vi "RWAllParameters_SRSI.vi"(8 "error in (no error)":errorcluster, 9 "Read/Write":T1(ring), 10 "Parameters In (Variant)":variant[](array[variant]), 11 "Parameters In":T2={"sensitivity"=0.11032028469750889, "Filter"={"Tau (fs)"=9.75e-13, "fwhm (fs)"=3.2551150895140684e-13, "filter gaussian power"=30}, "Poly Fit Order"=4, "N XPW Loop"=3, "Scales Unit"=enum."nm", "Results average"=0, "Spectral filter"={"min"=0.0, "max"=0.0, "Level"=0.0}, "Apodization"={"Auto"=TRUE, "WL min"=6.000000000000001e-07, "WL max"=1.0000000000000002e-06}, "Warning levels"={"Min level"=5000.0, "Max level"=62000.0, "Min contrast"=0.1}, "NormXPW"=FALSE, "DisableChecks"=FALSE, "External\nFund. Spectrum"=FALSE, "XPW factors"={"Optimize"=enum."Never", "Blue Shift Correction"=0.0, "Parasite Amp"=0.0}}) -> (0 "error out":errorcluster, 2 "Parameters Out":variant[](array[variant]), 3 "Parameters Out":T2={"sensitivity"=0.11032028469750889, "Filter"={"Tau (fs)"=9.75e-13, "fwhm (fs)"=3.2551150895140684e-13, "filter gaussian power"=30}, "Poly Fit Order"=4, "N XPW Loop"=3, "Scales Unit"=enum."nm", "Results average"=0, "Spectral filter"={"min"=0.0, "max"=0.0, "Level"=0.0}, "Apodization"={"Auto"=TRUE, "WL min"=6.000000000000001e-07, "WL max"=1.0000000000000002e-06}, "Warning levels"={"Min level"=5000.0, "Max level"=62000.0, "Min contrast"=0.1}, "NormXPW"=FALSE, "DisableChecks"=FALSE, "External\nFund. Spectrum"=FALSE, "XPW factors"={"Optimize"=enum."Never", "Blue Shift Correction"=0.0, "Parasite Amp"=0.0}})   [LabVIEW 2020]
uses:
  SRSI_Parameters.ctl
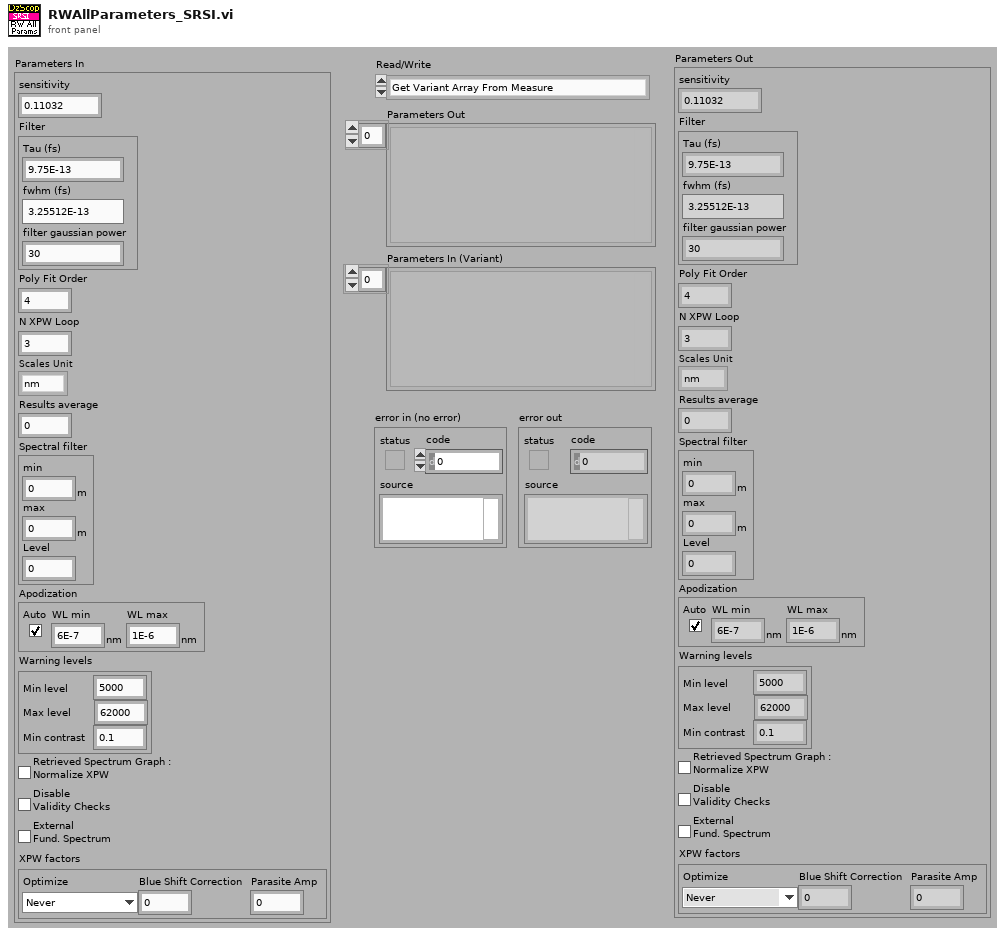
[diagram p1: front panel]
types:
  T1 = enum16{"Get Variant Array From Measure", "Set Measure From Variant Array"}
  T2 = typedef "SRSI_Parameters.ctl" = cluster{"sensitivity":dbl, "Filter":cluster{"Tau (fs)":dbl[unit], "fwhm (fs)":dbl[unit], "filter gaussian power":i32}, "Poly Fit Order":i32, "N XPW Loop":u16, "Scales Unit":enum16{"nm", "THz", "cm^-1"}, "Results average":i32, "Spectral filter":cluster{"min":dbl[unit], "max":dbl[unit], "Level":dbl}, "Apodization":cluster{"Auto":bool, "WL min":dbl[unit], "WL max":dbl[unit]}, "Warning levels":cluster{"Min level":dbl, "Max level":dbl, "Min contrast":dbl}, "NormXPW":bool, "DisableChecks":bool, "External\nFund. Spectrum":bool, "XPW factors":cluster{"Optimize":enum16{"Never", "Once", "Ever"}, "Blue Shift Correction":dbl, "Parasite Amp":dbl}}
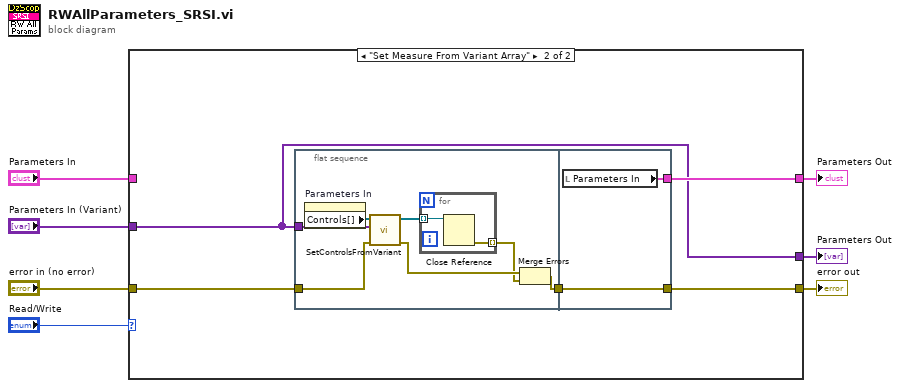
[diagram p0: block diagram]
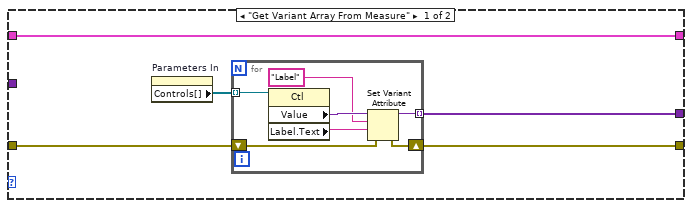
[diagram p2: hidden frame]
diagram:
  n1 = case shown="\"Set Measure From Variant Array\"" "Read/Write" {
    tunnel: "Parameters In" -> [w9 _]
    tunnel: [w10 w23] -> w3
    tunnel: "error in (no error)" -> [w12 w24]
    tunnel: [w11 w20] -> w4
    tunnel: "Parameters In (Variant)" -> [_ w20]
    tunnel: [w9 w21] -> w1
    frame "Get Variant Array From Measure" {
      n2 = property on="Parameters In" class="Clust (strict)"() -> ("Controls[]"=w8:refnum<vi>[])  [unwired: 2 in, 2 out]
      n3 = for {
        tunnel: w8 -> [w19] mode=indexing
        shift-right: [w16] -> w10
        shift-left: w12 -> [w17]
        tunnel: [w13] -> w11 mode=indexing
        n4 = property class="Ctl"(reference=w19) -> ("Value"=w18:variant, "Label.Text"=w15:string)  [unwired: 1 in, 2 out]
        n5 = Set Variant Attribute(Variant=w18, name="Label", value=w15, error in=w17) -> (Variant out=w13:variant, error out=w16:errorcluster)  [unwired: 1 out]
      }
    }
    frame "Set Measure From Variant Array" {
      n6 = flat-sequence {
        tunnel: w20 -> [w30]
        tunnel: w24 -> [w29]
        tunnel: [w27] -> w22
        tunnel: [w35] -> w23
        tunnel: w22 -> [w35]
        tunnel: [w34] -> w21
        frame #0 {
          n7 = property on="Parameters In" class="Clust (strict)"() -> ("Controls[]"=w31:refnum<vi>[])  [unwired: 2 in, 2 out]
          n8 = call "SetControlsFromVariant.vi"("error in"=w29, "Variant Array"=w30, "Controls[] in"=w31) -> ("error out"=w26:errorcluster, "Controls[] out"=w28:refnum<vi>[])  [unwired: 7 in]
          n9 = for {
            tunnel: w28 -> [w33] mode=indexing
            tunnel: [w32] -> w25 mode=indexing
            n10 = Close Reference(reference=w33) -> (error out=w32:errorcluster)  [unwired: 1 in]
          }
          n11 = Merge Errors(w26, w25) -> (w27:errorcluster)
        }
        frame #1 {
          n12 = local read "Parameters In"() -> (w34:T2)
        }
      }
    }
  }
  "error out" <- w3
  "Parameters Out" <- w1
  "Parameters Out" <- w4
